vi "CreateImagesv1.vi"() -> (3 "Images":T2)   [LabVIEW 2013]
uses:
  <vilib>/vision/Image Controls.llb/IMAQ Image.ctl
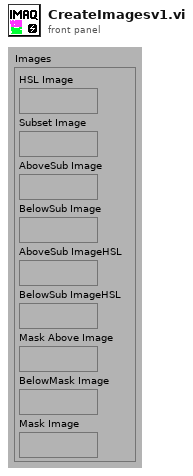
[diagram p1: front panel]
types:
  T1 = typedef "IMAQ Image.ctl" = refnum<image>
  T2 = cluster{"HSL Image":T1, "Subset Image":T1, "AboveSub Image":T1, "BelowSub Image":T1, "AboveSub ImageHSL":T1, "BelowSub ImageHSL":T1, "Mask Above Image":T1, "BelowMask Image":T1, "Mask Image":T1}
  T3 = typedef "Image Type" = u32
  T4 = cluster{"New Image":T1, "New Image":T1, "New Image":T1, "New Image":T1, "New Image":T1, "New Image":T1, "New Image":T1, "New Image":T1, "New Image":T1}
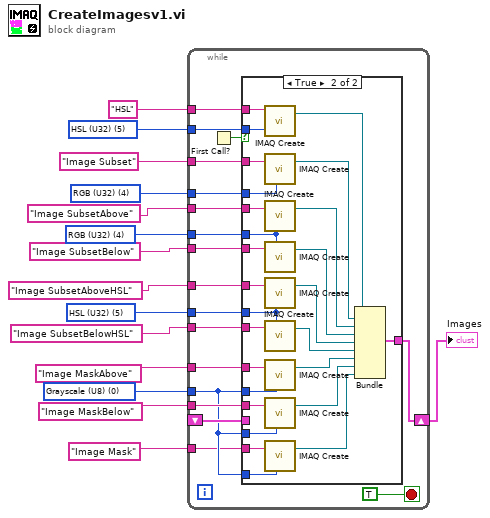
[diagram p0: block diagram]
diagram:
  w2 = T3 5 items=["Grayscale (U8)", "Grayscale (I16)", "Grayscale (SGL)", "Complex (CSG)", "RGB (U32)", "HSL (U32)", "RGB (U64)"] ("Image Type")
  w6 = T3 5 items=["Grayscale (U8)", "Grayscale (I16)", "Grayscale (SGL)", "Complex (CSG)", "RGB (U32)", "HSL (U32)", "RGB (U64)"] ("Image Type")
  w8 = T3 0 items=["Grayscale (U8)", "Grayscale (I16)", "Grayscale (SGL)", "Complex (CSG)", "RGB (U32)", "HSL (U32)", "RGB (U64)"] ("Image Type")
  w12 = T3 4 items=["Grayscale (U8)", "Grayscale (I16)", "Grayscale (SGL)", "Complex (CSG)", "RGB (U32)", "HSL (U32)", "RGB (U64)"] ("Image Type")
  w14 = T3 4 items=["Grayscale (U8)", "Grayscale (I16)", "Grayscale (SGL)", "Complex (CSG)", "RGB (U32)", "HSL (U32)", "RGB (U64)"] ("Image Type")
  n1 = while {
    tunnel: "Image Subset" ("Image Name") -> [w33]
    tunnel: w14 -> [w32]
    tunnel: "Image SubsetAbove" ("Image Name") -> [w31]
    tunnel: w12 -> [w30]
    tunnel: "Image SubsetBelow" ("Image Name") -> [w29]
    tunnel: "Image MaskAbove" ("Image Name") -> [w28]
    tunnel: "Image MaskBelow" ("Image Name") -> [w27]
    tunnel: w8 -> [w20]
    shift-right: [w26] -> w7
    shift-left: _ -> [w24]
    tunnel: w6 -> [w22]
    tunnel: "HSL" ("Image Name") -> [w21]
    tunnel: "Image Mask" ("Image Name") -> [w19]
    tunnel: w2 -> [w17]
    tunnel: "Image SubsetBelowHSL" ("Image Name") -> [w18]
    tunnel: "Image SubsetAboveHSL" ("Image Name") -> [w16]
    stop <- TRUE stop-if-true
    n2 = First Call?() -> (First Call?: T/F=w25:bool)
    n3 = case shown="True" w25 {
      tunnel: w33 -> [_ w60]
      tunnel: w32 -> [_ w59]
      tunnel: w31 -> [_ w58]
      tunnel: w30 -> [_ w57]
      tunnel: w29 -> [_ w56]
      tunnel: w28 -> [_ w55]
      tunnel: w27 -> [_ w54]
      tunnel: w20 -> [_ w53]
      tunnel: [w34 w49] -> w26
      tunnel: w20 -> [_ w48]
      tunnel: w24 -> [w34 _]
      tunnel: w22 -> [_ w47]
      tunnel: w21 -> [_ w46]
      tunnel: w20 -> [_ w44]
      tunnel: w19 -> [_ w43]
      tunnel: w16 -> [_ w40]
      tunnel: w17 -> [_ w41]
      tunnel: w18 -> [_ w42]
      frame False {
      }
      frame True {
        n4 = call "IMAQ Create"("Image Name"=w46, "Image Type"=w47) -> ("New Image"=w45:T1)  [unwired: 2 in, 2 out]
        n5 = call "IMAQ Create"("Image Name"=w60, "Image Type"=w59) -> ("New Image"=w50:T1)  [unwired: 2 in, 2 out]
        n6 = call "IMAQ Create"("Image Name"=w58, "Image Type"=w57) -> ("New Image"=w51:T1)  [unwired: 2 in, 2 out]
        n7 = call "IMAQ Create"("Image Name"=w56, "Image Type"=w57) -> ("New Image"=w52:T1)  [unwired: 2 in, 2 out]
        n8 = call "IMAQ Create"("Image Name"=w40, "Image Type"=w41) -> ("New Image"=w35:T1)  [unwired: 2 in, 2 out]
        n9 = call "IMAQ Create"("Image Name"=w42, "Image Type"=w41) -> ("New Image"=w36:T1)  [unwired: 2 in, 2 out]
        n10 = call "IMAQ Create"("Image Name"=w55, "Image Type"=w53) -> ("New Image"=w37:T1)  [unwired: 2 in, 2 out]
        n11 = call "IMAQ Create"("Image Name"=w54, "Image Type"=w48) -> ("New Image"=w38:T1)  [unwired: 2 in, 2 out]
        n12 = call "IMAQ Create"("Image Name"=w43, "Image Type"=w44) -> ("New Image"=w39:T1)  [unwired: 2 in, 2 out]
        n13 = Bundle("New Image"=w45, "New Image"=w50, "New Image"=w51, "New Image"=w52, "New Image"=w35, "New Image"=w36, "New Image"=w37, "New Image"=w38, "New Image"=w39) -> (w49:T4)  [unwired: 1 out]
      }
    }
  }
  "Images" <- w7
